vi "MCL Data Transactions List.vi"() -> (2 "Transactions":string[](array[string]))   [LabVIEW 2013]
uses:
  Names/Source Group Type.ctl
panel:
  in  "Sources":T1[](array[typedef])=[enum."LBCB1", enum."LBCB2", enum."Consolidated"]
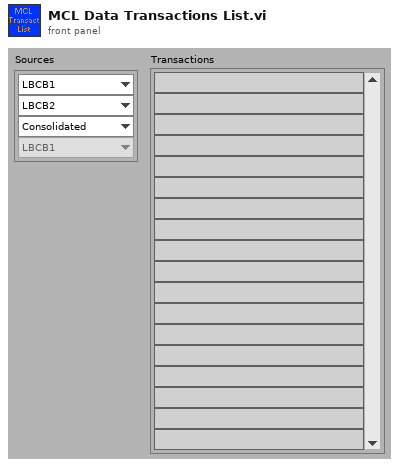
[diagram p1: front panel]
types:
  T1 = typedef "Source Group Type.ctl" = enum16{"LBCB1", "LBCB2", "Consolidated", "External"}
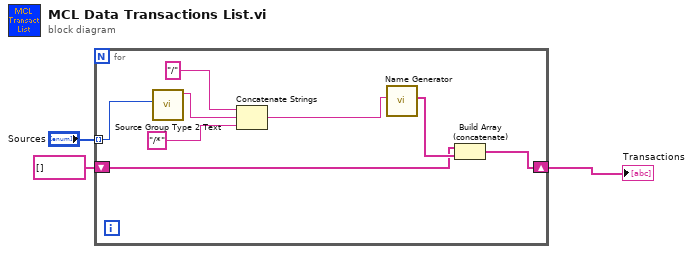
[diagram p0: block diagram]
diagram:
  n1 = for {
    tunnel: "Sources" -> [w11] mode=indexing
    shift-right: [w5] -> w2
    shift-left: string[] [] -> [w4]
    n2 = call "Source Group Type 2 Text.vi"("Source"=w11) -> ("String"=w10:string)  [unwired: 10 in]
    n3 = Concatenate Strings("/" ("string"), w10, "/*" ("string")) -> (w7:string)
    n4 = call "Name Generator.vi"("Group Specifier"=w7) -> ("Group Names"=w6:string[])  [unwired: 10 in]
    n5 = Build Array (concatenate)(w4, w6) -> (w5:string[])
  }
  "Transactions" <- w2
